vi "Add Expt Device.vi"(8 "error in (no error)":errorcluster, 10 "Expt Device Details":string[](array[string]), 11 "Experiment Name":string) -> (0 "error out":errorcluster)   [LabVIEW 2011]
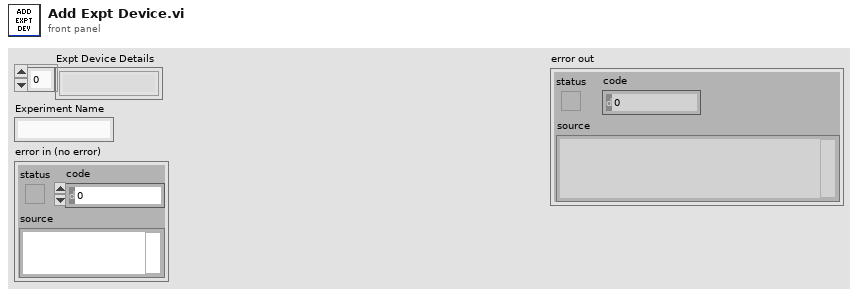
[diagram p1: front panel]
types:
  T1 = typedef "mysql_authentication.ctl" = cluster{"User":string, "Password":string, "Database":string}
  T2 = cluster{"Port":u16, "IP Address":string, "Authentication":T1}
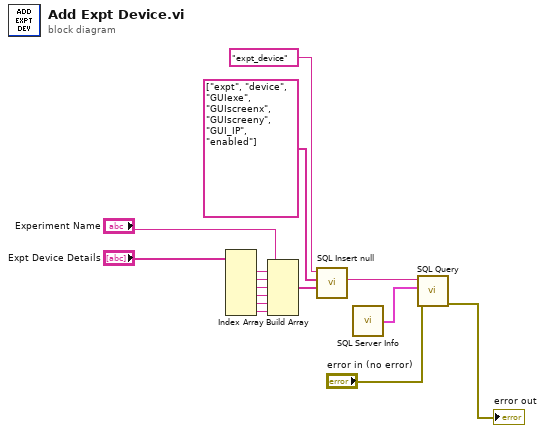
[diagram p0: block diagram]
diagram:
  n1 = Index Array(array="Expt Device Details") -> (element #1=w10:string, element #2=w9:string, element #3=w8:string, element #4=w7:string, element #5=w6:string, element #6=w5:string)  [unwired: 6 in]
  n2 = Build Array("Experiment Name", w10, w9, w8, w7, w6, w5) -> (w12:string[])
  n3 = call "SQL Insert null.vi"("Values"=w12, "Column Names"=string[] ["expt", "device", "GUIexe", "GUIscreenx", "GUIscreeny", "GUI_IP", "enabled"] ("Field Names"), "Table"="expt_device") -> ("Query String"=w13:string)  [unwired: 8 in]
  n4 = call "SQL Server Info.vi"() -> ("SQL Server Info"=w3:T2)
  n5 = call "SQL Query.vi"("error in (no error)"="error in (no error)", "SQL Server Info"=w3, "Query"=w13) -> ("error out"=→"error out":errorcluster)  [unwired: 7 in, 1 out]
